vi "Update SciScan Objective Info with OME data.vi"(8 "error in (no error)":errorcluster, 11 "Objective Parameters":T1[](array[typedef])) -> (0 "error out":errorcluster)   [LabVIEW 2012]
doc: "SciScan 1.2 160622"
uses:
  Custom Controls and Typedefs/Objective Parameters Cluster.ctl
  GFG/GFGfpRefGet.vi
  GFG/GFG library.lvlib
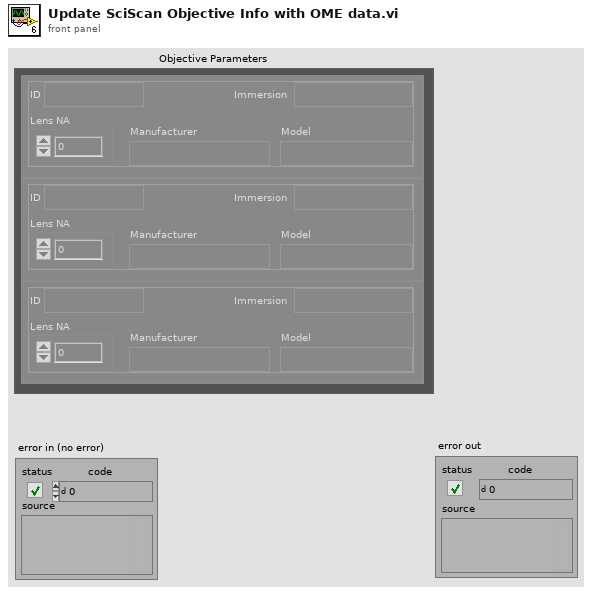
[diagram p1: front panel]
types:
  T1 = typedef "Objective Parameters Cluster.ctl" = cluster{"ID":string, "Immersion":string, "Lens NA":dbl, "Manufacturer":string, "Model":string}
  T2 = cluster{"WaveformChartRef":refnum<vi>, "DigitalRef":refnum<vi>, "ArrayRef":refnum<vi>, "TabControlRef":refnum<vi>, "EnumRef":refnum<vi>, "RingRef":refnum<vi>, "BooleanRef":refnum<vi>, "KnobRef":refnum<vi>, "SlideRef":refnum<vi>, "PathRef":refnum<vi>, "StringRef":refnum<vi>, "ComboBox":refnum<vi>, "WaveformGraphRef":refnum<vi>}
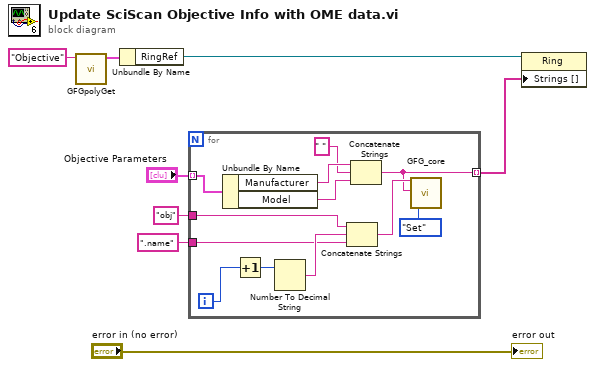
[diagram p0: block diagram]
diagram:
  n1 = call-poly "GFGpolyGet.vi"("Variable Name in"="Objective") -> ("output cluster"=w8:T2)  [unwired: 9 in, 1 out]
  n2 = Unbundle By Name(w8) -> ("RingRef"=w2:refnum<vi>)
  n3 = for {
    tunnel: "Objective Parameters" -> [w20] mode=indexing
    tunnel: "obj" ("Variable Name in") -> [w16]
    tunnel: ".name" ("Variable Name in") -> [w15]
    tunnel: [w9] -> w3 mode=indexing
    i -> [w17]
    n4 = Unbundle By Name(w20) -> ("Manufacturer"=w12:string, "Model"=w11:string)
    n5 = Increment(x=w17) -> (x+1=w18:i32)
    n6 = Number To Decimal String(number=w18) -> (decimal integer string=w19:string)  [unwired: 1 in]
    n7 = Concatenate Strings(w16, w19, w15) -> (w13:string)
    n8 = Concatenate Strings(w12, " " ("string"), w11) -> (w9:string)
    n9 = call "GFG_core.vi"("Variable Name in"=w13, "Variant in"=w9, "Action"=enum16{"Init", "Set", "Get", "Clear"}."Set") -> ()  [unwired: 10 in, 7 out]
  }
  n10 = property class="Ring"(reference=w2, "Strings []"=w3) -> ()  [unwired: 1 in, 2 out]
  "error out" <- "error in (no error)"
